vi "Open_2_Rtoom.vi"(7 "error in (no error)":errorcluster, 10 "Motor Settings":T1={"Left Motor"={"Inversion"=TRUE, "PWM Channel"=enum."PWM 0"}, "Right Motor"={"Inversion"=TRUE, "PWM Channel"=enum."PWM 1"}}) -> (0 "error out":errorcluster, 3 "RobotDriveDevRef":T3={"DevStatus"={"status"=FALSE, "code"=0, "source"=""}, "Motors[]"=[], "Square Inputs"=FALSE, "Max Output"=1.0})   [LabVIEW 2018]
doc: "Opens a reference to the robot drive for a four-motor robot using Rev Robotics SPARK motor controllers.\n\nThis software is licensed. Open the labview\\readme\\WPI Robotics Library Open Source License.txt file for more information."
uses:
  <vilib>/Rock Robotics/WPI/RobotDrive/WPI_RobotDriveDevRef.ctl
  <vilib>/Rock Robotics/WPI/MotorControl/WPI_MotorControlDeviceRef.ctl
  <vilib>/Rock Robotics/WPI/MotorControl/WPI_MotorControlType.ctl
  <vilib>/Rock Robotics/SystemInterfaces/DIO/FPGA_DIOPWMChannel.ctl
  <vilib>/Rock Robotics/WPI/PWM/WPI_PWMDeadband.ctl
  <vilib>/Rock Robotics/SystemInterfaces/DIO/FPGA_DIOChannel.ctl
  Intake/Implementation/Intake Motor Settings.ctl
  <vilib>/Rock Robotics/WPI/SafetyOutput/WPI_SafetyOutputConfigMenu.ctl
  <vilib>/Rock Robotics/WPI/MotorControl/WPI_MotorControlOpen SPARK.vi
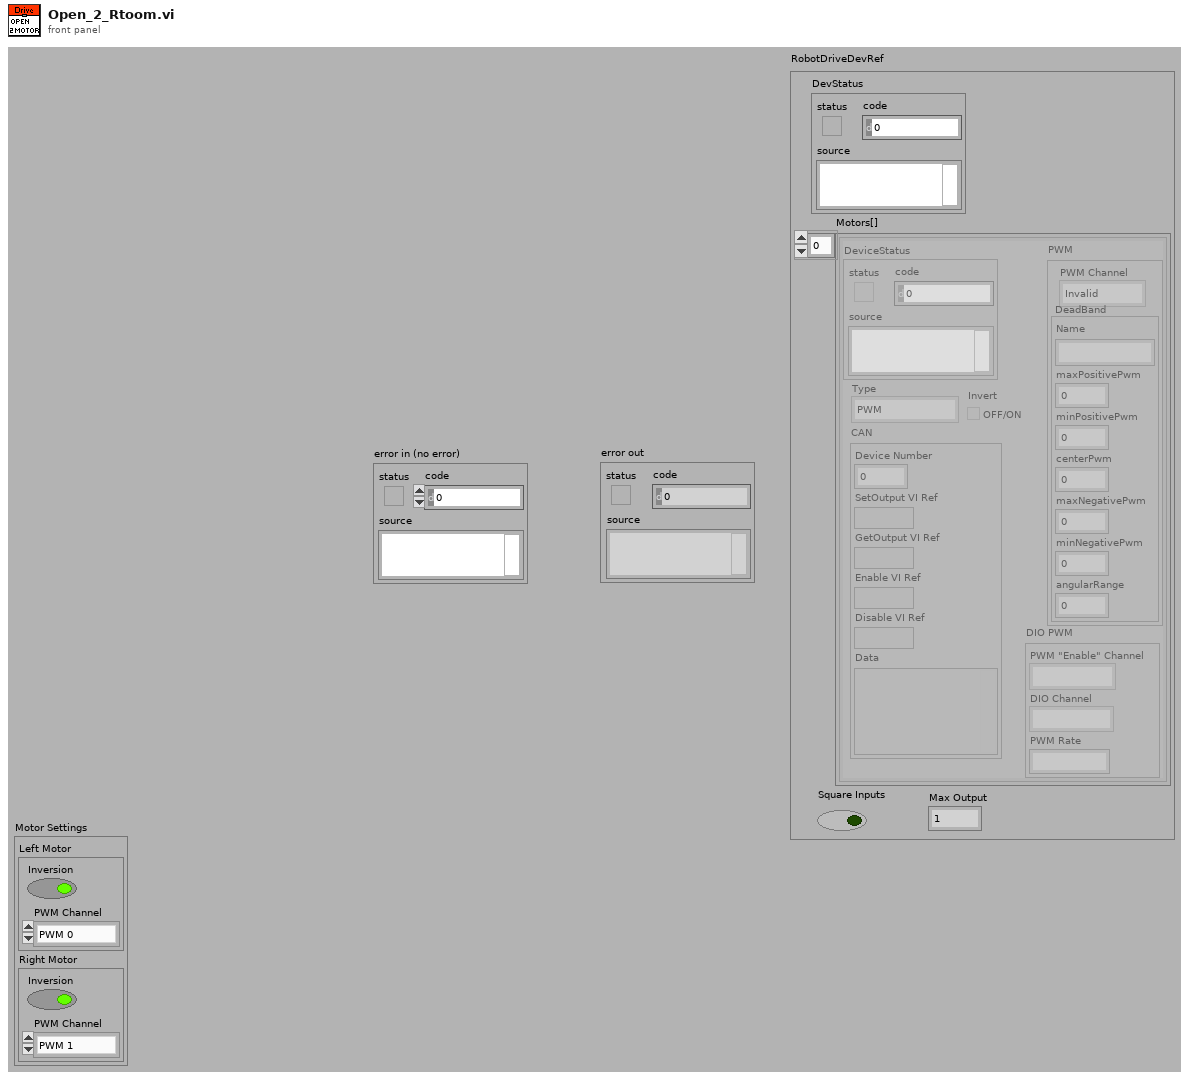
[diagram p1: front panel]
types:
  T1 = typedef "Intake Motor Settings.ctl" = cluster{"Left Motor":cluster{"Inversion":bool, "PWM Channel":T2}, "Right Motor":cluster{"Inversion":bool, "PWM Channel":T2}}
  T2 = typedef "FPGA_DIOPWMChannel.ctl" = enum8{"PWM 0", "PWM 1", "PWM 2", "PWM 3", "PWM 4", "PWM 5", "PWM 6", "PWM 7", "PWM 8", "PWM 9", "PWM MXP 0", "PWM MXP 1", "PWM MXP 2", "PWM MXP 3", "PWM MXP 4", "PWM MXP 5", "PWM MXP 6", "PWM MXP 7", "PWM MXP 8", "PWM MXP 9", "Invalid"}
  T3 = typedef "WPI_RobotDriveDevRef.ctl" = cluster{"DevStatus":errorcluster, "Motors[]":T4[], "Square Inputs":bool, "Max Output":dbl}
  T4 = typedef "WPI_MotorControlDeviceRef.ctl" = cluster{"DeviceStatus":errorcluster, "Type":T5, "PWM":cluster{"PWM Channel":T2, "DeadBand":T6}, "CAN":cluster{"Device Number":u8, "SetOutput VI Ref":variant, "GetOutput VI Ref":variant, "Enable VI Ref":variant, "Disable VI Ref":variant, "Data":variant}, "Invert":bool, "DIO PWM":cluster{"PWM \"Enable\" Channel":T2, "DIOChannel":T7, "PWM Rate":dbl}}
  T5 = typedef "WPI_MotorControlType.ctl" = enum16{"PWM", "CAN", "DIO PWM"}
  T6 = typedef "WPI_PWMDeadband.ctl" = cluster{"Name":string, "maxPositivePwm":i32, "minPositivePwm":i32, "centerPwm":i32, "maxNegativePwm":i32, "minNegativePwm":i32, "angularRange":u16}
  T7 = typedef "FPGA_DIOChannel.ctl" = enum8{"DIO 0", "DIO 1", "DIO 2", "DIO 3", "DIO 4", "DIO 5", "DIO 6", "DIO 7", "DIO 8", "DIO 9", "DIO MXP 0", "DIO MXP 1", "DIO MXP 2", "DIO MXP 3", "DIO MXP 4", "DIO MXP 5", "DIO MXP 6", "DIO MXP 7", "DIO MXP 8", "DIO MXP 9", "DIO MXP 10", "DIO MXP 11", "DIO MXP 12", "DIO MXP 13", "DIO MXP 14", "DIO MXP 15", "SPI Port CS1", "SPI Port CS2", "SPI Port CS3", "SPI Port MISO", "SPI Port MOSI", "Invalid"}
  T8 = typedef "WPI_SafetyOutputConfigMenu.ctl" = enum16{"Enable", "Disable"}
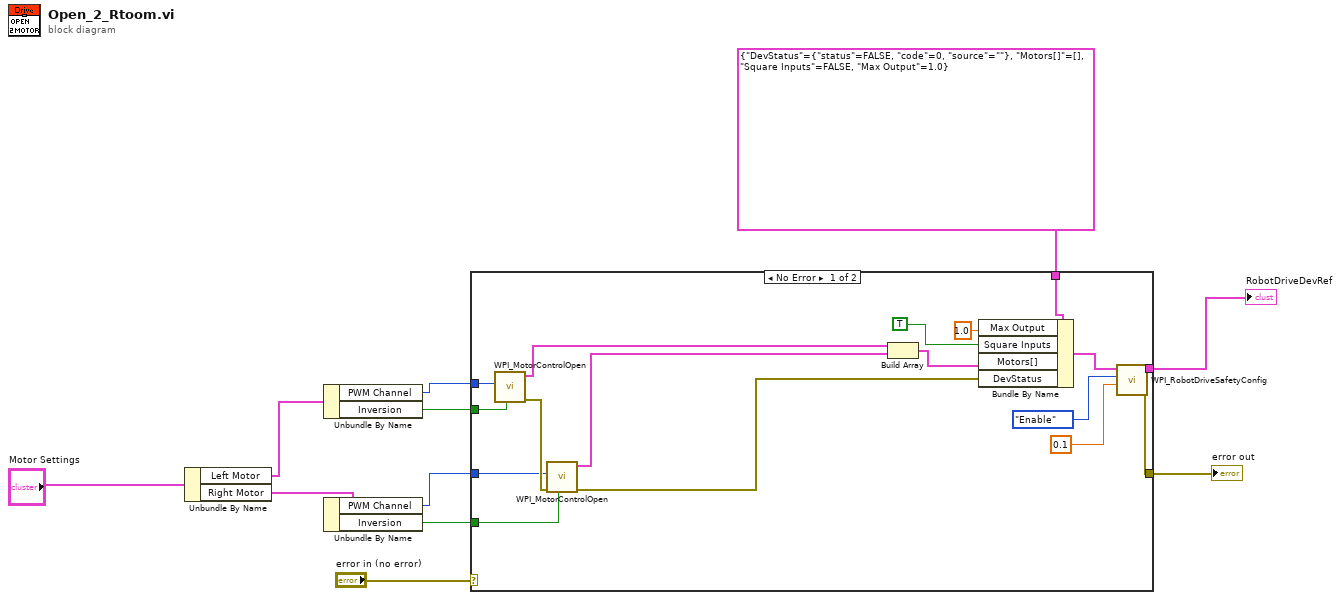
[diagram p0: block diagram]
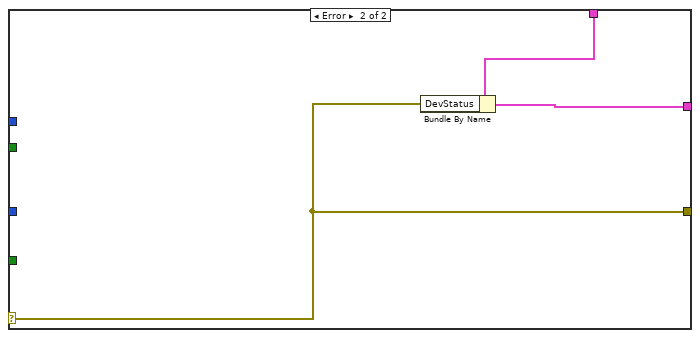
[diagram p2: hidden frame]
diagram:
  n1 = Unbundle By Name("Motor Settings") -> ("Left Motor"=w7:cluster{"Inversion":bool, "PWM Channel":T2}, "Right Motor"=w6:cluster{"Inversion":bool, "PWM Channel":T2})
  n2 = Unbundle By Name(w7) -> ("PWM Channel"=w5:T2, "Inversion"=w4:bool)
  n3 = Unbundle By Name(w6) -> ("PWM Channel"=w3:T2, "Inversion"=w2:bool)
  n4 = case shown="No Error" "error in (no error)" {
    selector: "error in (no error)" -> [_ w29]
    tunnel: [w19 w30] -> w11
    tunnel: T3 {"DevStatus"={"status"=FALSE, "code"=0, "source"=""}, "Motors[]"=[], "Square Inputs"=FALSE, "Max Output"=1.0} ("RobotDriveDevRef") -> [w28 w31]
    tunnel: [w20 w29] -> w8
    tunnel: w5 -> [w16 _]
    tunnel: w4 -> [w15 _]
    tunnel: w3 -> [w14 _]
    tunnel: w2 -> [w13 _]
    frame No Error {
      n5 = call-poly <vilib>:"WPI_MotorControlOpen.vi"("Invert"=w15, "PWM Channel"=w16) -> ("error out"=w24:errorcluster, "MotorControlDeviceRef"=w26:T4)  [unwired: 2 in, 6 out]
      n6 = call-poly <vilib>:"WPI_MotorControlOpen.vi"("Invert"=w13, "error in (no error)"=w24, "PWM Channel"=w14) -> ("error out"=w12:errorcluster, "MotorControlDeviceRef"=w25:T4)  [unwired: 1 in, 6 out]
      n7 = Build Array(w26, w25) -> (w23:T4[])
      n8 = Bundle By Name(cluster=w28, "Max Output"=1.0, "Square Inputs"=TRUE ("DestroyPWM?"), "Motors[]"=w23, "DevStatus"=w12) -> (w21:T3)
      n9 = call <vilib>:"WPI_RobotDriveSafetyConfig.vi"("timeout (s)"=0.1, "mode"=WPI_SafetyOutputConfigMenu."Enable", "RobotDriveDevRef"=w21) -> ("error out"=w20:errorcluster, "RobotDriveDevRef"=w19:T3)  [unwired: 1 in, 6 out]
    }
    frame Error {
      n10 = Bundle By Name(cluster=w31, "DevStatus"=w29) -> (w30:T3)
    }
  }
  "RobotDriveDevRef" <- w11
  "error out" <- w8
